vi "escribe_ tbl_ra_generador_ext.vi"(6 "id_pon_frecuencia":i32, 7 "last_id_ajuste_previo":string, 8 "error in (no error)":errorcluster, 9 "usuario_registra":i32, 10 "Tabla Referencia Acústica Generador Externo":string[][](table), 11 "BD in":refnum<class "Base de Datos.lvclass">) -> (0 "error out":errorcluster, 3 "BD out":refnum<class "Base de Datos.lvclass">)   [LabVIEW 2019, in "Base de Datos.lvclass"]
uses:
  Base de Datos.lvclass
  Base de Datos.lvclass/Base de Datos.ctl
  SQLiteConnector/SQLiteConnection.lvclass
panel:
  out "Paso 2":string
  # "Tabla que registra los datos de referencia Acústica Generador Externo"
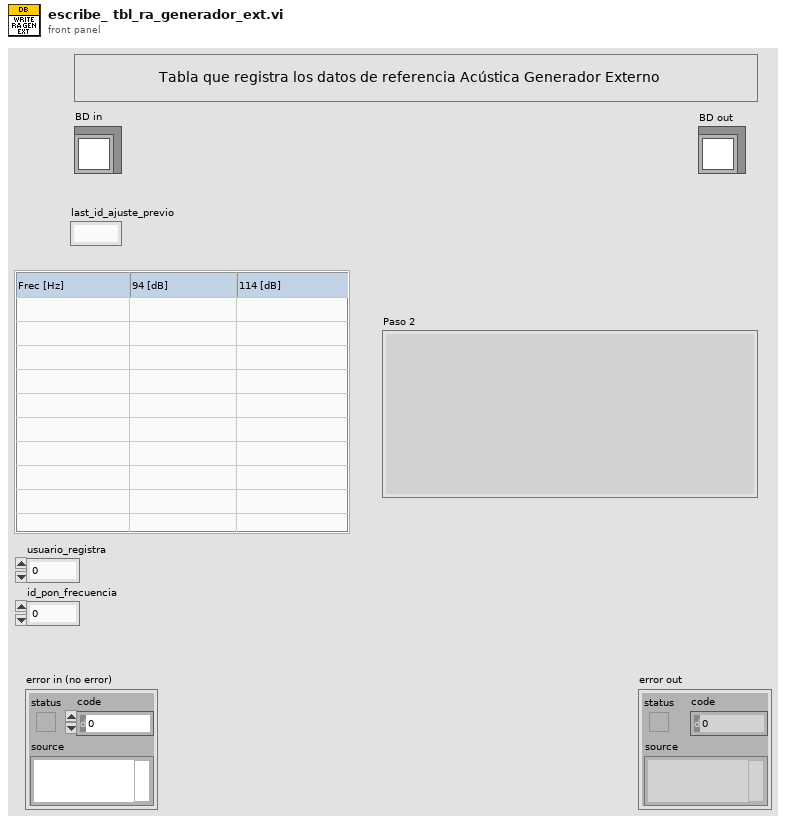
[diagram p1: front panel]
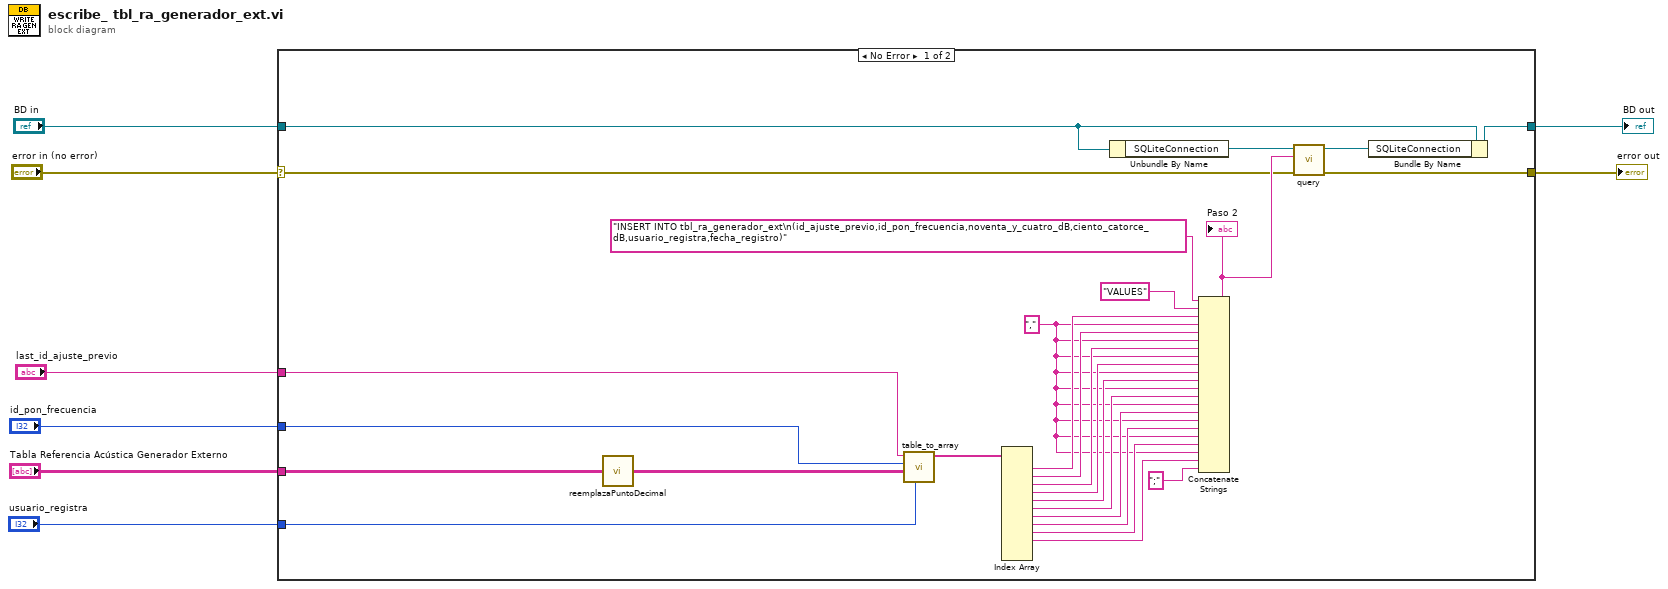
[diagram p0: block diagram]
diagram:
  n1 = case shown="No Error" "error in (no error)" {
    selector: "error in (no error)" -> [w16 w37]
    tunnel: [w35 w37] -> w8
    tunnel: "Tabla Referencia Acústica Generador Externo" -> [w10 _]
    tunnel: "id_pon_frecuencia" -> [w18 _]
    tunnel: "usuario_registra" -> [w17 _]
    tunnel: "BD in" -> [w13 w36]
    tunnel: "last_id_ajuste_previo" -> [w15 _]
    tunnel: [w12 w36] -> w1
    frame No Error {
      w22 = "," ("string")
      n2 = call "reemplazaPuntoDecimal.vi"("Tabla Referencia Acústica Generador Externo in"=w10) -> ("Tabla Referencia Acústica Generador Externo out"=w9:string[][])
      n3 = call "table_to_array.vi"("usuario_registra"=w17, "Tabla Referencia Acústica Generador Externo"=w9, "id_pon_frecuencia"=w18, "last_id_ajuste_previo"=w15) -> ("Array"=w32:string[])  [unwired: 6 in, 1 out]
      n4 = Index Array(array=w32) -> (element #1=w31:string, element #2=w30:string, element #3=w29:string, element #4=w28:string, element #5=w27:string, element #6=w26:string, element #7=w25:string, element #8=w24:string, element #9=w23:string, element #10=w21:string)  [unwired: 12 in, 2 out]
      n5 = Unbundle By Name(w13) -> ("SQLiteConnection"=w14:refnum<class "SQLiteConnection.lvclass">)
      n6 = Concatenate Strings("INSERT INTO tbl_ra_generador_ext\n(id_ajuste_previo,id_pon_frecuencia,noventa_y_cuatro_dB,ciento_catorce_dB,usuario_registra,fecha_registro)" ("format string"), "VALUES" ("string"), w31, w22, w30, w22, w29, w22, w28, w22, w27, w22, w26, w22, w25, w22, w24, w22, w23, w22, w21, ";" ("string")) -> (w19:string)
      "Paso 2" <- w19
      n7 = call "query.vi"("error in (no error)"=w16, "SQL Statement"=w19, "object in"=w14) -> ("error out"=w35:errorcluster, "object out"=w11:refnum<class "SQLiteConnection.lvclass">)  [unwired: 5 in, 2 out]
      n8 = Bundle By Name(cluster=w13, "SQLiteConnection"=w11) -> (w12:refnum<class "Base de Datos.lvclass">)
    }
    frame Error {
    }
  }
  "error out" <- w8
  "BD out" <- w1
